vi "Climber Controller.vi"(8 "error in":errorcluster) -> ()   [LabVIEW 2017]
doc: "This VI executes continuously carrying out the current operation and responding to updates or new operations. It will often contain the timing or control code that is difficult to place directly in TeleOp. This VI generally opens all sensors and motors and isolates the rest of the robot code from knowing how the operations are carried out."
uses:
  Climber Setpoints.ctl
  Climber Operations.ctl
  Users/Public/Documents/Cross The Road Electronics/Phoenix-LabVIEW/Motor Controller/Controls/CTRE_Phoenix_MotorControl_ControlMode.ctl
  <vilib>/Rock Robotics/WPI/ThirdParty/Phoenix-LabVIEW/Motor Controller/Controls/CTRE_Phoenix_MotorControl_NeutralMode.ctl
  <vilib>/Rock Robotics/WPI/Solenoid/WPI_SolenoidChannel.ctl
  <vilib>/Rock Robotics/WPI/Solenoid/WPI_SolenoidValue.ctl
  <vilib>/Rock Robotics/WPI/Solenoid/WPI_SolenoidSetEnum.vi
  <vilib>/Rock Robotics/WPI/Solenoid/WPI_SolenoidOpenSingle.vi
  <vilib>/Rock Robotics/Network Tables/NT Write Boolean.vi
panel:
  out "Current\nCmd":string
  # "Tip: It may be helpful to observe inputs and sensor values.\nYou may also want to display tuning or debugging controls."
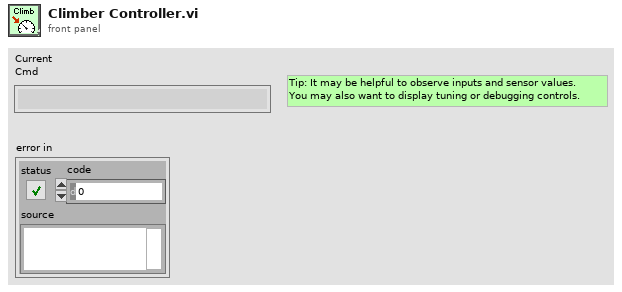
[diagram p1: front panel]
types:
  T1 = typedef "WPI_SolenoidChannel.ctl" = enum8{"Solenoid 0", "Solenoid 1", "Solenoid 2", "Solenoid 3", "Solenoid 4", "Solenoid 5", "Solenoid 6", "Solenoid 7", "Invalid"}
  T2 = typedef "CTRE_Phoenix_MotorControl_NeutralMode.ctl" = enum8{"EEPROMSetting", "Override to Coast", "Override to Brake"}
  T3 = typedef "CTRE_Phoenix_MotorControl_ControlMode.ctl" = u16
  T4 = typedef "Climber Setpoints.ctl" = cluster{"Operation":T5, "Climber Speed":dbl, "Duration":dbl}
  T5 = typedef "Climber Operations.ctl" = enum16{"Reserve", "Read Current", "Climb"}
  T6 = typedef "WPI_MotorControlDeviceRef.ctl" = cluster{"DeviceStatus":errorcluster, "Type":T7, "PWM":cluster{"PWM Channel":T8, "DeadBand":T9}, "CAN":cluster{"Device Number":u8, "SetOutput VI Ref":variant, "GetOutput VI Ref":variant, "Enable VI Ref":variant, "Disable VI Ref":variant, "Data":variant}, "Invert":bool, "DIO PWM":cluster{"PWM \"Enable\" Channel":T8, "DIOChannel":T10, "PWM Rate":dbl}}
  T7 = typedef "WPI_MotorControlType.ctl" = enum16{"PWM", "CAN", "DIO PWM"}
  T8 = typedef "FPGA_DIOPWMChannel.ctl" = enum8{"PWM 0", "PWM 1", "PWM 2", "PWM 3", "PWM 4", "PWM 5", "PWM 6", "PWM 7", "PWM 8", "PWM 9", "PWM MXP 0", "PWM MXP 1", "PWM MXP 2", "PWM MXP 3", "PWM MXP 4", "PWM MXP 5", "PWM MXP 6", "PWM MXP 7", "PWM MXP 8", "PWM MXP 9", "Invalid"}
  T9 = typedef "WPI_PWMDeadband.ctl" = cluster{"Name":string, "maxPositivePwm":i32, "minPositivePwm":i32, "centerPwm":i32, "maxNegativePwm":i32, "minNegativePwm":i32, "angularRange":u16}
  T10 = typedef "FPGA_DIOChannel.ctl" = enum8{"DIO 0", "DIO 1", "DIO 2", "DIO 3", "DIO 4", "DIO 5", "DIO 6", "DIO 7", "DIO 8", "DIO 9", "DIO MXP 0", "DIO MXP 1", "DIO MXP 2", "DIO MXP 3", "DIO MXP 4", "DIO MXP 5", "DIO MXP 6", "DIO MXP 7", "DIO MXP 8", "DIO MXP 9", "DIO MXP 10", "DIO MXP 11", "DIO MXP 12", "DIO MXP 13", "DIO MXP 14", "DIO MXP 15", "SPI Port CS1", "SPI Port CS2", "SPI Port CS3", "SPI Port MISO", "SPI Port MOSI", "Invalid"}
  T11 = typedef "WPI_SolenoidDevRef.ctl" = cluster{"DevStatus":errorcluster, "Pneumatics Control Module":u8, "Forward Solenoid Channel":T1, "Reverse Solenoid Channel":T1}
  T12 = typedef "Command Status Info.ctl" = cluster{"Name":string, "Status":T13, "notifier out":T14}
  T13 = typedef "Completion Status.ctl" = enum16{"Successful", "Aborted", "Incomplete"}
  T14 = typedef "Completion Notifier.ctl" = refnum<notifier>
  T15 = cluster{"Default Command":T4, "Command Timing":cluster{"Start Time (ms)":u32, "Iterations":i32}, "Command Arguments":cluster{"Command Info":T12, "Description":string, "Default Command":T4, "notifier out":refnum<notifier>, "Subsystem Name":string}}
  T16 = typedef "WPI_SolenoidValue.ctl" = enum16{"Off", "On", "Forward", "Reverse"}
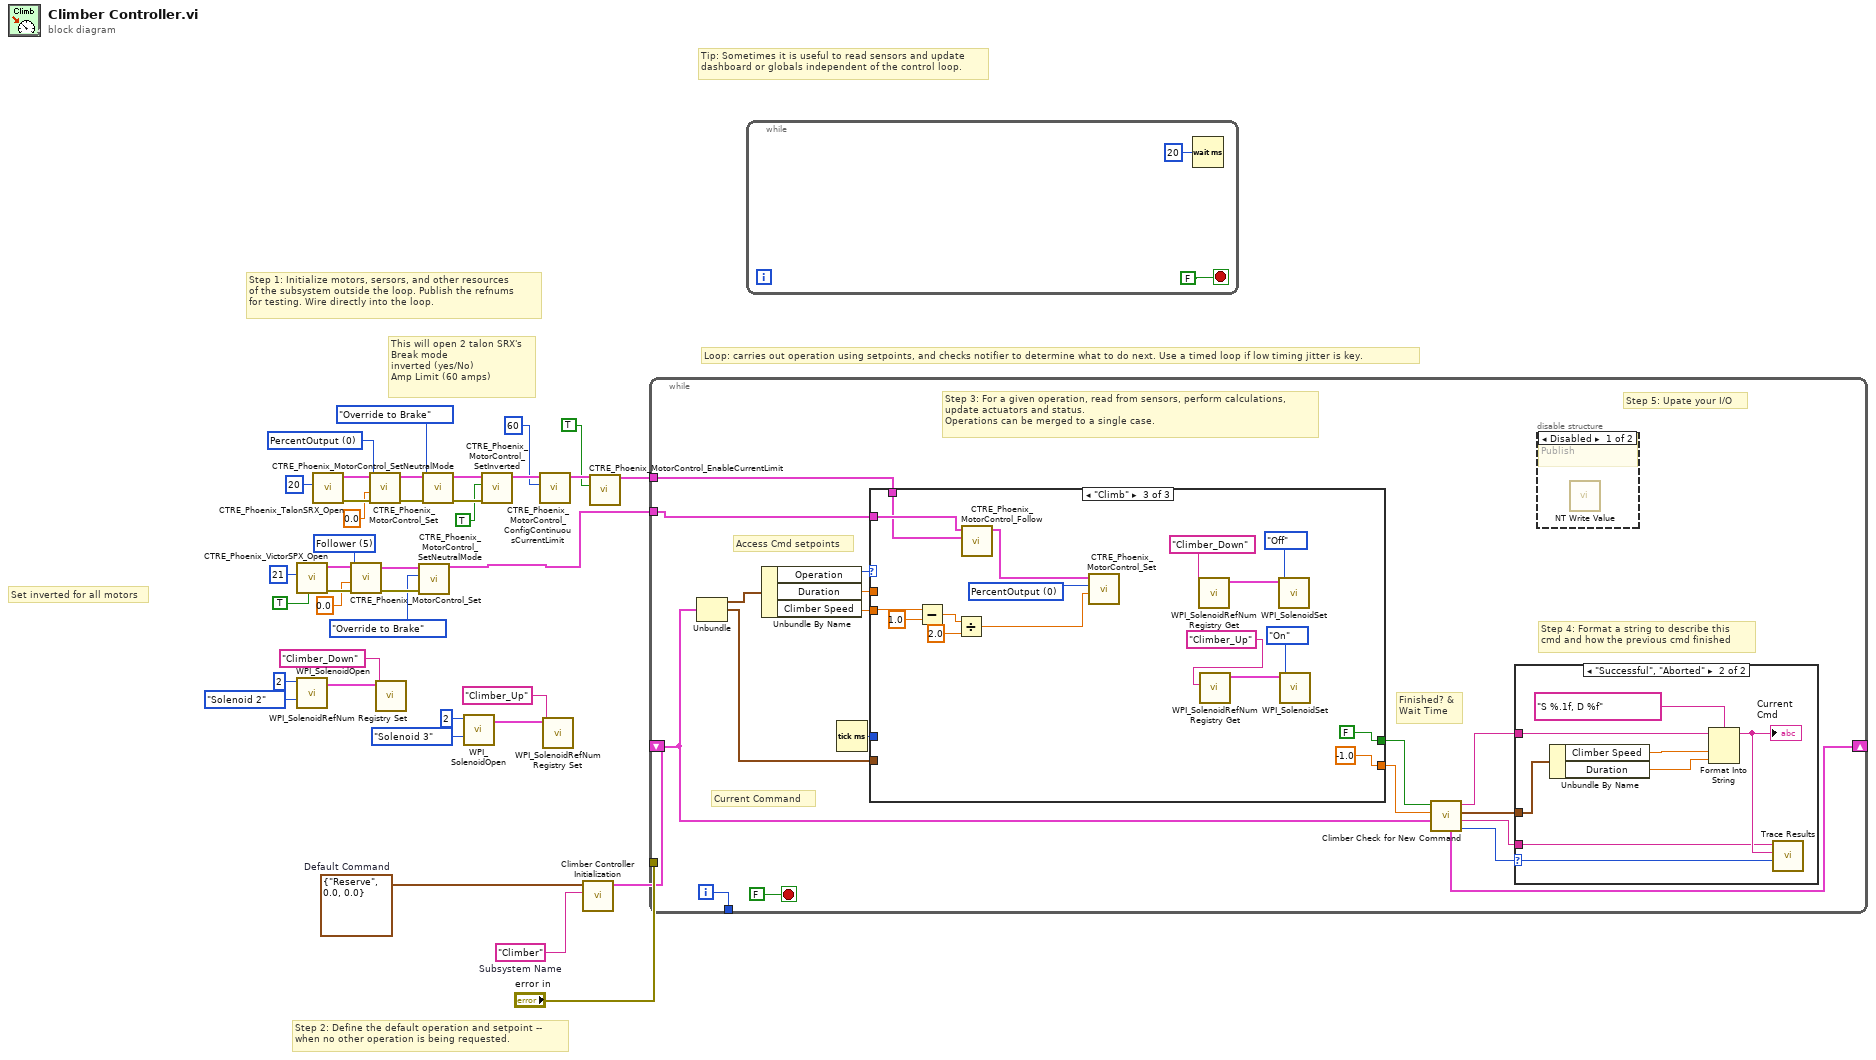
[diagram p0: block diagram]
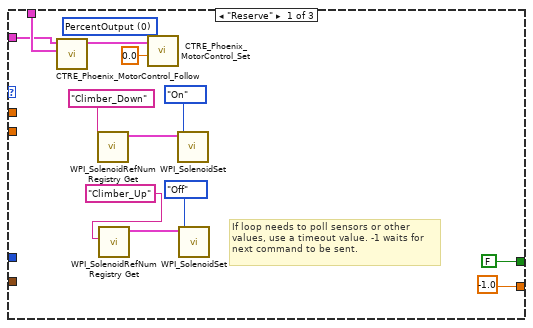
[diagram p4: hidden frame]
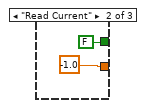
[diagram p5: hidden frame]
diagram:
  w20 = T3 5 items=["PercentOutput"=0, "Position"=1, "Velocity"=2, "Follower"=5, "MotionProfile"=6, "MotionMagic"=7, "MotionMagicArc"=8, "TimedPercentOutput"=9, "Disabled"=15] ("Control Mode")
  w32 = T3 0 items=["PercentOutput"=0, "Position"=1, "Velocity"=2, "Follower"=5, "MotionProfile"=6, "MotionMagic"=7, "MotionMagicArc"=8, "TimedPercentOutput"=9, "Disabled"=15] ("Control Mode")
  w35 = T4 {"Operation"=enum."Reserve", "Climber Speed"=0.0, "Duration"=0.0}  # Default Command
  w36 = "Climber"  # Subsystem Name
  # "This will open 2 talon SRX's\nBreak mode\ninverted (yes/No)\nAmp Limit (60 amps)"
  # "Set inverted for all motors"
  # "Tip: Sometimes it is useful to read sensors and update\ndashboard or globals independent of the control loop."
  # "Step 2: Define the default operation and setpoint --\nwhen no other operation is being requested."
  # "Step 1: Initialize motors, sersors, and other resources\nof the subsystem outside the loop. Publish the refnums\nfor testing. Wire directly into the loop."
  # "Loop: carries out operation using setpoints, and checks notifier to determine what to do next. Use a timed loop if low timing jitter is key."
  n1 = call <vilib>:"CTRE_Phoenix_VictorSPX_Open.vi"("Invert"=TRUE, "Device Number"=u8 21) -> ("error out"=w22:errorcluster, "CAN Talon SRX Ref"=w21:T6)  [unwired: 8 in]
  n2 = call-poly <vilib>:"WPI_SolenoidOpen.vi"("Solenoid Channel"=WPI_SolenoidChannel."Solenoid 2", "Pneumatics Control Module (0)"=u8 2) -> ("SolenoidDevRef"=w9:T11)  [unwired: 8 in, 1 out]
  n3 = call <vilib>:"CTRE_Phoenix_TalonSRX_Open.vi"("Device Number"=u8 20) -> ("error out"=w34:errorcluster, "CAN Talon SRX Ref"=w33:T6)  [unwired: 9 in]
  n4 = call <vilib>:"CTRE_Phoenix_MotorControl_Set.vi"("error in (no error)"=w22, "Output"=0.0, "Control Mode"=w20, "PhoenixMotorControlDevRef"=w21) -> ("error out"=w11:errorcluster, "PhoenixMotorControlDevRef"=w12:T6)  [unwired: 6 in]
  n5 = call <vilib>:"CTRE_Phoenix_MotorControl_Set.vi"("error in (no error)"=w34, "Output"=0.0, "Control Mode"=w32, "PhoenixMotorControlDevRef"=w33) -> ("error out"=w29:errorcluster, "PhoenixMotorControlDevRef"=w28:T6)  [unwired: 6 in]
  n6 = call <vilib>:"WPI_SolenoidRefNum Registry Set.vi"("refnum name"="Climber_Down", "SolenoidDevRef"=w9) -> ()  [unwired: 8 in, 2 out]
  n7 = call <vilib>:"CTRE_Phoenix_MotorControl_SetNeutralMode.vi"("error in (no error)"=w11, "Motor Control Neutral Mode"=CTRE_Phoenix_MotorControl_NeutralMode."Override to Brake", "PhoenixMotorControlDevRef"=w12) -> ("PhoenixMotorControlDevRef"=w1:T6)  [unwired: 7 in, 1 out]
  n8 = call <vilib>:"CTRE_Phoenix_MotorControl_SetNeutralMode.vi"("error in (no error)"=w29, "Motor Control Neutral Mode"=CTRE_Phoenix_MotorControl_NeutralMode."Override to Brake", "PhoenixMotorControlDevRef"=w28) -> ("error out"=w26:errorcluster, "PhoenixMotorControlDevRef"=w25:T6)  [unwired: 7 in]
  n9 = call-poly <vilib>:"WPI_SolenoidOpen.vi"("Solenoid Channel"=WPI_SolenoidChannel."Solenoid 3", "Pneumatics Control Module (0)"=u8 2) -> ("SolenoidDevRef"=w5:T11)  [unwired: 8 in, 1 out]
  n10 = call <vilib>:"CTRE_Phoenix_MotorControl_SetInverted.vi"("error in (no error)"=w26, "Invert?"=TRUE, "PhoenixMotorControlDevRef"=w25) -> ("PhoenixMotorControlDevRef"=w17:T6)  [unwired: 7 in, 1 out]
  n11 = call <vilib>:"CTRE_Phoenix_MotorControl_ConfigContinuousCurrentLimit.vi"("Continuous Current Limit (Amps)"=60, "PhoenixMotorControlDevRef"=w17) -> ("PhoenixMotorControlDevRef"=w15:T6)  [unwired: 8 in, 1 out]
  n12 = call <vilib>:"WPI_SolenoidRefNum Registry Set.vi"("refnum name"="Climber_Up", "SolenoidDevRef"=w5) -> ()  [unwired: 8 in, 2 out]
  n13 = call "Climber Controller Initialization.vi"("Subsystem Name"=w36, "Default Command"=w35) -> ("Command Info"=w37:T15)  [unwired: 9 in]
  n14 = call <vilib>:"CTRE_Phoenix_MotorControl_EnableCurrentLimit.vi"("Enable Current Limit?"=TRUE, "PhoenixMotorControlDevRef"=w15) -> ("PhoenixMotorControlDevRef"=w13:T6)  [unwired: 8 in, 1 out]
  n15 = while {
    shift-right: [w47] -> _
    shift-left: w37 -> [w48]
    tunnel: [w55] -> _
    tunnel: "error in" -> [_]
    tunnel: w13 -> [w40]
    tunnel: w1 -> [w39]
    i -> [w55]
    stop <- FALSE stop-if-true
    # "Step 5: Upate your I/O"
    # "Step 4: Format a string to describe this\ncmd and how the previous cmd finished"
    # "Current Command"
    # "Access Cmd setpoints"
    # "Finished? &\nWait Time"
    # "Step 3: For a given operation, read from sensors, perform calculations,\nupdate actuators and status.\nOperations can be merged to a single case."
    n16 = Unbundle(w48) -> ("Default Command"=w54:T4, "Command Timing"=w50:cluster{"Start Time (ms)":u32, "Iterations":i32})  [unwired: 1 out]
    n17 = Unbundle By Name(w54) -> ("Operation"=w53:T5, "Duration"=w52:dbl, "Climber Speed"=w49:dbl)
    n18 = Tick Count (ms)() -> (millisecond timer value=w51:u32)
    n19 = case shown="\"Climb\"" w53 {
      tunnel: [-1.0 -1.0 -1.0] -> w45
      tunnel: [FALSE ("ignore previous (F)") FALSE ("ignore previous (F)") FALSE ("ignore previous (F)")] -> w46
      tunnel: w50 -> [_ _ _]
      tunnel: w52 -> [_ _ _]
      tunnel: w51 -> [_ _ _]
      tunnel: w49 -> [_ _ w94]
      tunnel: w40 -> [w69 _ w83]
      tunnel: w39 -> [w68 _ w84]
      frame "Reserve" {
        w66 = T3 0 items=["PercentOutput"=0, "Position"=1, "Velocity"=2, "Current"=3, "Follower"=5, "MotionProfile"=6, "MotionMagic"=7, "MotionMagicArc"=8, "MotionProfileArc"=10, "Disabled"=15] ("Control Mode")
        # "If loop needs to poll sensors or other\nvalues, use a timeout value. -1 waits for\nnext command to be sent."
        n20 = call <vilib>:"CTRE_Phoenix_MotorControl_Follow.vi"("Master Controller to Follow"=w69, "PhoenixMotorControlDevRef"=w68) -> ("PhoenixMotorControlDevRef"=w67:T6)  [unwired: 8 in, 1 out]
        n21 = call <vilib>:"WPI_SolenoidRefNum Registry Get.vi"("refnum name"="Climber_Down") -> ("SolenoidDevRef"=w75:T11)  [unwired: 9 in, 1 out]
        n22 = call <vilib>:"WPI_SolenoidRefNum Registry Get.vi"("refnum name"="Climber_Up") -> ("SolenoidDevRef"=w72:T11)  [unwired: 9 in, 1 out]
        n23 = call <vilib>:"CTRE_Phoenix_MotorControl_Set.vi"("Output"=0.0, "Control Mode"=w66, "PhoenixMotorControlDevRef"=w67) -> ()  [unwired: 7 in, 2 out]
        n24 = call-poly <vilib>:"WPI_SolenoidSet.vi"("Value"=WPI_SolenoidValue."On", "SolenoidDevRef"=w75) -> ()  [unwired: 8 in, 2 out]
        n25 = call-poly <vilib>:"WPI_SolenoidSet.vi"("Value"=WPI_SolenoidValue."Off", "SolenoidDevRef"=w72) -> ()  [unwired: 8 in, 2 out]
      }
      frame "Read Current" {
      }
      frame "Climb" {
        w80 = T3 0 items=["PercentOutput"=0, "Position"=1, "Velocity"=2, "Current"=3, "Follower"=5, "MotionProfile"=6, "MotionMagic"=7, "MotionMagicArc"=8, "MotionProfileArc"=10, "Disabled"=15] ("Control Mode")
        n26 = Subtract(x=w94, y=1.0) -> (x-y=w92:dbl)
        n27 = Divide(x=w92, y=2.0) -> (x/y=w81:dbl)
        n28 = call <vilib>:"CTRE_Phoenix_MotorControl_Follow.vi"("Master Controller to Follow"=w83, "PhoenixMotorControlDevRef"=w84) -> ("PhoenixMotorControlDevRef"=w82:T6)  [unwired: 8 in, 1 out]
        n29 = call <vilib>:"CTRE_Phoenix_MotorControl_Set.vi"("Output"=w81, "Control Mode"=w80, "PhoenixMotorControlDevRef"=w82) -> ()  [unwired: 7 in, 2 out]
        n30 = call <vilib>:"WPI_SolenoidRefNum Registry Get.vi"("refnum name"="Climber_Down") -> ("SolenoidDevRef"=w90:T11)  [unwired: 9 in, 1 out]
        n31 = call <vilib>:"WPI_SolenoidRefNum Registry Get.vi"("refnum name"="Climber_Up") -> ("SolenoidDevRef"=w87:T11)  [unwired: 9 in, 1 out]
        n32 = call-poly <vilib>:"WPI_SolenoidSet.vi"("Value"=WPI_SolenoidValue."Off", "SolenoidDevRef"=w90) -> ()  [unwired: 8 in, 2 out]
        n33 = call-poly <vilib>:"WPI_SolenoidSet.vi"("Value"=WPI_SolenoidValue."On", "SolenoidDevRef"=w87) -> ()  [unwired: 8 in, 2 out]
      }
    }
    n34 = call "Climber Check for New Command.vi"("Current Command"=w48, "Wait time (ms)"=w45, "Finished?"=w46) -> ("Completion"=w41:T13, "Subsystem Name"=w42:string, "Current Command"=w43:T4, "Initial Trace String"=w44:string, "NextCommand"=w47:T15)  [unwired: 4 in]
    n35 = case shown="\"Successful\", \"Aborted\"" w41 {
      selector: w41 -> [_ w64]
      tunnel: w44 -> [_ w60]
      tunnel: w43 -> [_ w61]
      tunnel: w42 -> [_ w57]
      frame "Incomplete", Default {
        # "Continuing current command"
      }
      frame "Successful", "Aborted" {
        # "Report and setup for next command"
        n36 = Unbundle By Name(w61) -> ("Climber Speed"=w63:dbl, "Duration"=w58:dbl)
        n37 = Format Into String(format string="S %.1f, D %f", initial string=w60, w63, w58) -> (resulting string=w59:string)  [unwired: 1 in, 1 out]
        "Current\nCmd" <- w59
        n38 = call <vilib>:"Trace Results.vi"("Status of previous command"=w64, "Description"=w59, "Subsystem"=w57) -> ()  [unwired: 9 in]
      }
    }
    n39 = disable-structure shown="Disabled" {
      frame Disabled {
        # "Publish"
        n40 = call-poly <vilib>:"NT Write Value.vi"() -> ()  [unwired: 11 in, 1 out]
      }
      frame Enabled {
      }
    }
  }
  n41 = while {
    stop <- FALSE stop-if-true
    n42 = Wait (ms)(milliseconds to wait=u32 20) -> ()  [unwired: 1 out]
  }
